vi "Check Application MUXList.vi"(8 "error in (no error)":errorcluster, 10 "Source":string, 11 "SLSC Switch in":refnum<class "SLSC Switch.lvclass">) -> (0 "error out":errorcluster, 1 "Destinations":string[](array[string]), 2 "found?":bool, 3 "SLSC Switch out":refnum<class "SLSC Switch.lvclass">, 4 "index":i32)   [LabVIEW 2015, in "SLSC Switch.lvlib" / "SLSC Switch.lvclass"]
uses:
  SLSC Switch.lvclass
  SLSC Switch.lvclass/SLSC Switch.ctl
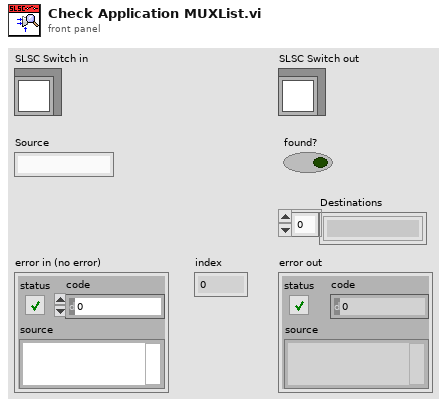
[diagram p1: front panel]
types:
  T1 = typedef "SLSC Switch.lvlib/SLSC Switch.lvclass/MuxList Entry.ctl" = cluster{"Source":string, "Destinations":string[]}
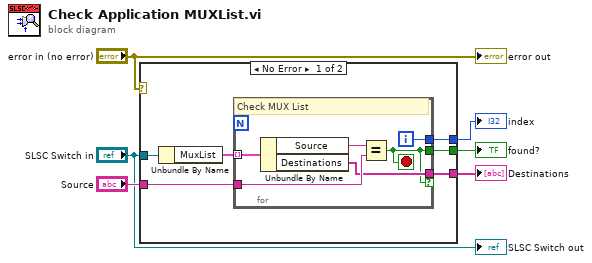
[diagram p0: block diagram]
diagram:
  n1 = case shown="No Error" "error in (no error)" {
    tunnel: "Source" -> [w12 _]
    tunnel: "SLSC Switch in" -> [w11 _]
    tunnel: [w10 _] -> w4
    tunnel: [w8 _] -> w3
    tunnel: [w7 _] -> w1
    frame No Error {
      n2 = Unbundle By Name(w11) -> ("MuxList"=w9:T1[])
      n3 = for {
        tunnel: w12 -> [w18]
        tunnel: w9 -> [w17] mode=indexing
        tunnel: [w15] -> w7
        tunnel: [w13] -> w10
        tunnel: [w14] -> w8 if=w13
        i -> [w15]
        stop <- w13 stop-if-true
        # "Check MUX List"
        n4 = Unbundle By Name(w17) -> ("Source"=w16:string, "Destinations"=w14:string[])
        n5 = Equal?(x=w16, y=w18) -> (x = y?=w13:bool)
      }
    }
    frame Error {
    }
  }
  "found?" <- w4
  "Destinations" <- w3
  "index" <- w1
  "SLSC Switch out" <- "SLSC Switch in"
  "error out" <- "error in (no error)"
